vi "getDelay.vi"(8 "error in (no error)":errorcluster, 11 "Instrument.DelayLine in":refnum<class "Instrument.DelayLine.lvclass">) -> (0 "error out":errorcluster, 2 "delay (ps)":dbl, 3 "Instrument.DelayLine out":refnum<class "Instrument.DelayLine.lvclass">, 4 "Finished?":bool)   [LabVIEW 2019, in "Instrument.DelayLine.lvclass"]
uses:
  Instrument.DelayLine.lvclass
  C:/Users/patrick/Documents/GitHub/Instrument-Framework/lvsrc/Framework/Instrument/Instrument.lvclass
  Typedefs/DelayLine.Commands--Enum.ctl
  58737b40-2911-4442-99f6-99a085f4d414.vi
  58737b40-2911-4442-99f6-99a085f4d414.vi/b7290ad0-2231-43b0-b29d-9614a8be47cb.vi
  58737b40-2911-4442-99f6-99a085f4d414.vi/678f7225-7165-494e-bb21-9d9c04622572.vi
  <vilib>/Utility/Data Type/Get Type Information.vi
  <vilib>/JDP Science/JSONtext/JSON text to Variant.vi
  <vilib>/JDP Science/JSONtext/LVClass Serializer/JSONtext LVClass Serializer.lvclass
  Instrument/Instrument.lvclass
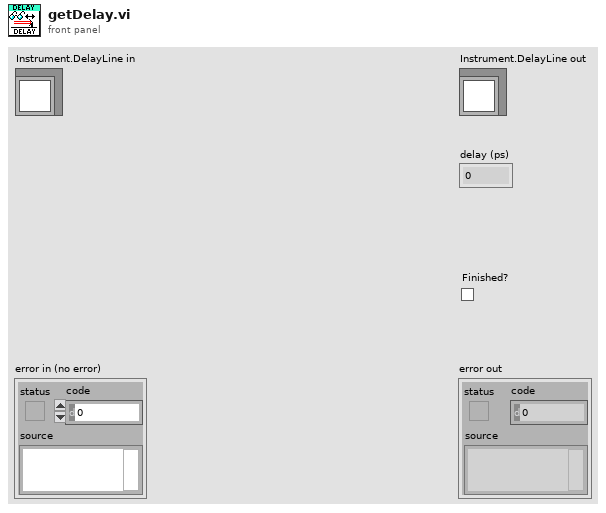
[diagram p1: front panel]
types:
  T1 = typedef "Instrument.DelayLine.lvclass/DelayLine.Commands--Enum.ctl" = enum16{"getDelay", "setDelay"}
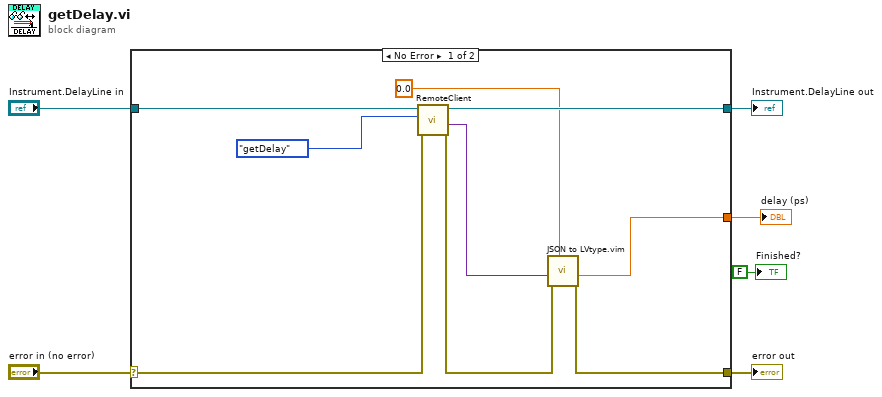
[diagram p0: block diagram]
diagram:
  n1 = case shown="No Error" "error in (no error)" {
    selector: "error in (no error)" -> [w12 w17]
    tunnel: [w10 w17] -> w5
    tunnel: [w15 w16] -> w3
    tunnel: "Instrument.DelayLine in" -> [w14 w16]
    tunnel: [w7 _] -> w2
    frame No Error {
      n2 = call "RemoteClient.vi"("error in (no error)"=w12, "Command in"=DelayLine.Commands--Enum."getDelay" ("command"), "Instrument in"=w14) -> ("error out"=w11:errorcluster, "Data out"=w9:variant, "Instrument out"=w15:refnum<class "Instrument.DelayLine.lvclass">)  [unwired: 5 in, 1 out]
      n3 = call "JSON to LVtype.vim"("type"=0.0, "error in (no error)"=w11, "JSON Data in"=w9) -> ("error out"=w10:errorcluster, "Data out"=w7:dbl)  [unwired: 7 in]
    }
    frame Error {
    }
  }
  "error out" <- w5
  "Instrument.DelayLine out" <- w3
  "delay (ps)" <- w2
  "Finished?" <- FALSE ("Finished?")
